vi "Get Authentication Encryption.vi"(8 "error in (no error)":errorcluster, 11 "SSID":string) -> (0 "error out":errorcluster, 2 "Encryption":string, 3 "Authentication":string)   [LabVIEW 2017]
doc: "Returns the authentication and encryption type. Special cases are defined as Microsoft did not consistently use some labels in netsh and XML."
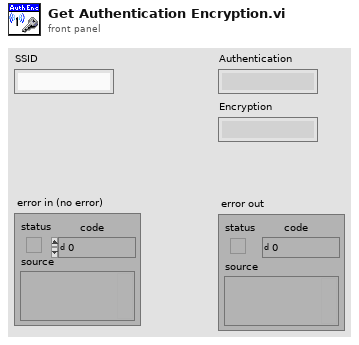
[diagram p1: front panel]
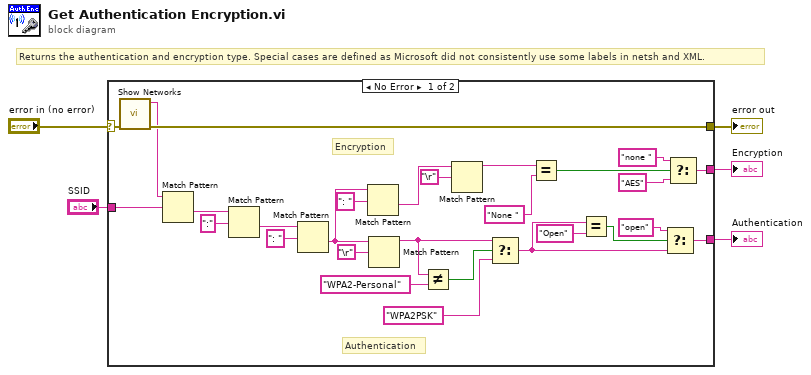
[diagram p0: block diagram]
diagram:
  # "Returns the authentication and encryption type. Special cases are defined as Microsoft did not consistently use some labels in netsh and XML."
  n1 = case shown="No Error" "error in (no error)" {
    selector: "error in (no error)" -> [w8 w34]
    tunnel: [w7 w34] -> w4
    tunnel: "SSID" -> [w16 _]
    tunnel: [w9 _] -> w2
    tunnel: [w15 _] -> w1
    frame No Error {
      # "Authentication"
      # "Encryption"
      n2 = call "Show Networks.vi"("error in (no error)"=w8) -> ("error out"=w7:errorcluster, "Feedback"=w6:string)  [unwired: 8 in, 1 out]
      n3 = Match Pattern(string=w6, regular expression=w16) -> (after substring=w31:string)  [unwired: 1 in, 3 out]
      n4 = Match Pattern(string=w31, regular expression=":" ("string")) -> (after substring=w29:string)  [unwired: 1 in, 3 out]
      n5 = Match Pattern(string=w29, regular expression=": " ("string")) -> (after substring=w24:string)  [unwired: 1 in, 3 out]
      n6 = Match Pattern(string=w24, regular expression=": ") -> (after substring=w21:string)  [unwired: 1 in, 3 out]
      n7 = Match Pattern(string=w24, regular expression="\r") -> (before substring=w27:string)  [unwired: 1 in, 3 out]
      n8 = Not Equal?(x=w27, y="WPA2-Personal") -> (x != y?=w25:bool)
      n9 = Match Pattern(string=w21, regular expression="\r") -> (before substring=w12:string)  [unwired: 1 in, 3 out]
      n10 = Select(t=w27, s=w25, f="WPA2PSK") -> (s? t:f=w17:string)
      n11 = Equal?(x=w12, y="None " ("regular expression")) -> (x = y?=w11:bool)
      n12 = Equal?(x=w17, y="Open") -> (x = y?=w19:bool)
      n13 = Select(t="open" ("y"), s=w19, f=w17) -> (s? t:f=w15:string)
      n14 = Select(t="none " ("regular expression"), s=w11, f="AES" ("regular expression")) -> (s? t:f=w9:string)
    }
    frame Error {
    }
  }
  "error out" <- w4
  "Authentication" <- w1
  "Encryption" <- w2
